vi "licdf app encrypt.vi"(0 "handle":i32, 1 "out":string, 2 "out_len":i32, 5 "scope":i32, 7 "plaintext":string, 9 "plaintext_len":i32, 11 "error in (no error)":errorcluster, 12 "out_cap":i32) -> (3 "out out":string, 4 "out_len out":i32, 6 "function return":i32, 15 "error out":errorcluster)   [LabVIEW 2026, in "keynub_licdongle.lvlib"]
doc: "int32_t licdf_app_encrypt(int32_t handle, int32_t scope, const uint8_t *plaintext,\n int32_t plaintext_len, uint8_t *out, int32_t out_cap,\n int32_t *out_len);"
uses:
  keynub_licdongle.lvlib
  natives/win-x64/keynub_licdongle_flat.dll
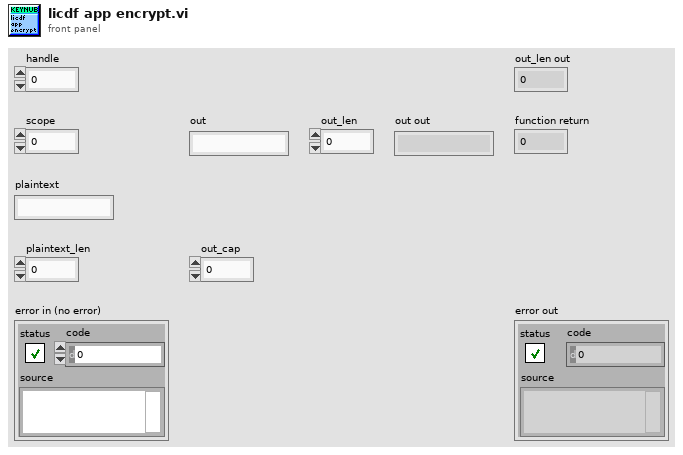
[diagram p1: front panel]
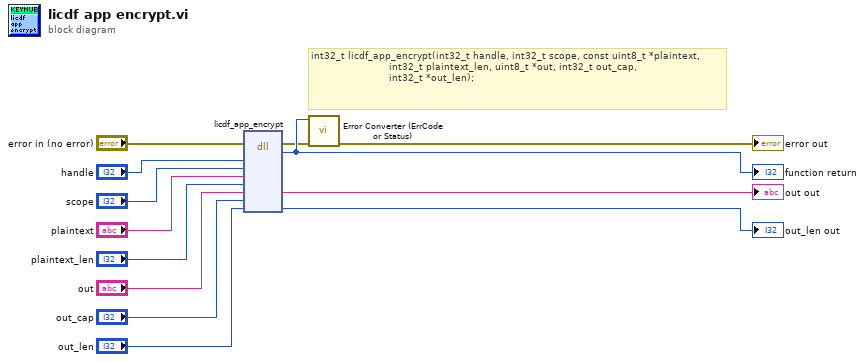
[diagram p0: block diagram]
diagram:
  # "int32_t licdf_app_encrypt(int32_t handle, int32_t scope, const uint8_t *plaintext,\n                          int32_t plaintext_len, uint8_t *out, int32_t out_cap,\n                          int32_t *out_len);"
  n1 = dll-call lib="C:/Austausch/KeyNub/LicenseDongle-PublicSDK/natives/win-x64/keynub_licdongle_flat.*" fn="licdf_app_encrypt"(error in="error in (no error)", "handle"="handle", "scope"="scope", "plaintext"="plaintext", "plaintext_len"="plaintext_len", "out"="out", "out_cap"="out_cap", "out_len"="out_len") -> (error out=w2:errorcluster, w13:i32, "out"=→"out out":string, "out_len"=→"out_len out":i32)  [unwired: 7 in, 1 out]
  "function return" <- w13
  n2 = call "Error Converter (ErrCode or Status).vi"("error in (no error)"=w2, "error code"=w13) -> ("error out"=→"error out":errorcluster)  [unwired: 9 in]
